vi "Get protocol behavior.vi"(1 "Protocol":T1) -> (0 "RT Management.lvlib:FTP.lvclass":refnum<class "File Transfer Behavior.lvclass">)   [LabVIEW 2015, in "Tests.lvlib"]
uses:
  Tests.lvlib
  Protocol.ctl
  classes/File Transfer Behavior/File Transfer Behavior.lvclass
  classes/WebDAV/WebDAV.lvclass
  classes/FTP/FTP.lvclass
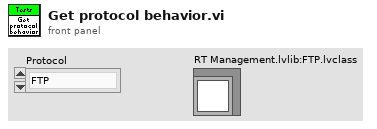
[diagram p1: front panel]
types:
  T1 = typedef "Tests.lvlib/Protocol.ctl" = enum16{"FTP", "WebDAV"}
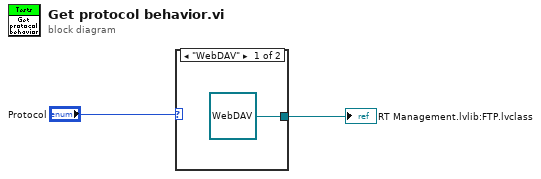
[diagram p0: block diagram]
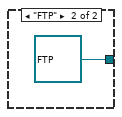
[diagram p2: hidden frame]
diagram:
  n1 = case shown="\"WebDAV\"" "Protocol" {
    tunnel: [refnum<class "WebDAV.lvclass"> refnum ("RT Management.lvlib:WebDAV.lvclass") refnum<class "FTP.lvclass"> refnum ("RT Management.lvlib:FTP.lvclass")] -> w1
    frame "WebDAV" {
    }
    frame "FTP" {
    }
  }
  "RT Management.lvlib:FTP.lvclass" <- w1
